vi "getFPGAWriteTimeout.vi"(11 "Modbus in":refnum<class "Modbus.lvclass">) -> (2 "FPGAWriteTimeout":i32=10, 3 "Modbus out":refnum<class "Modbus.lvclass">)   [LabVIEW 2015]
uses:
  Modbus.lvclass
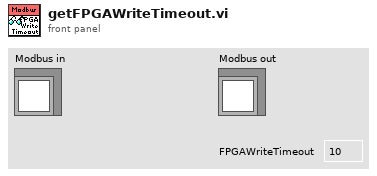
[diagram p1: front panel]
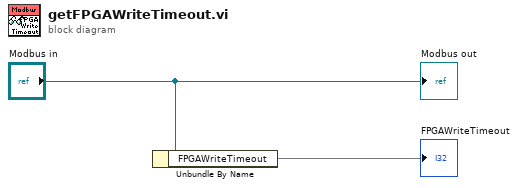
[diagram p0: block diagram]
diagram:
  n1 = Unbundle By Name("Modbus in") -> ("FPGAWriteTimeout"=→"FPGAWriteTimeout")
  "Modbus out" <- "Modbus in"
